vi "LM79 Stabilization.vi"(8 "error in (no error)":errorcluster, 10 "Time Between\nMeasurements (s)":dbl, 11 "Data over time":dbl[](array[numeric])) -> (0 "error out":errorcluster, 1 "Stabilization Data":T1, 2 "Stabilized":bool)   [LabVIEW 2013]
uses:
  MR 16 teardown/MR16TestStandDAQ/Controls/Stabilization.ctl
  <vilib>/Analysis/baseanly.llb/Mean (DBL).vi
  <vilib>/Analysis/NI_AALBase.lvlib
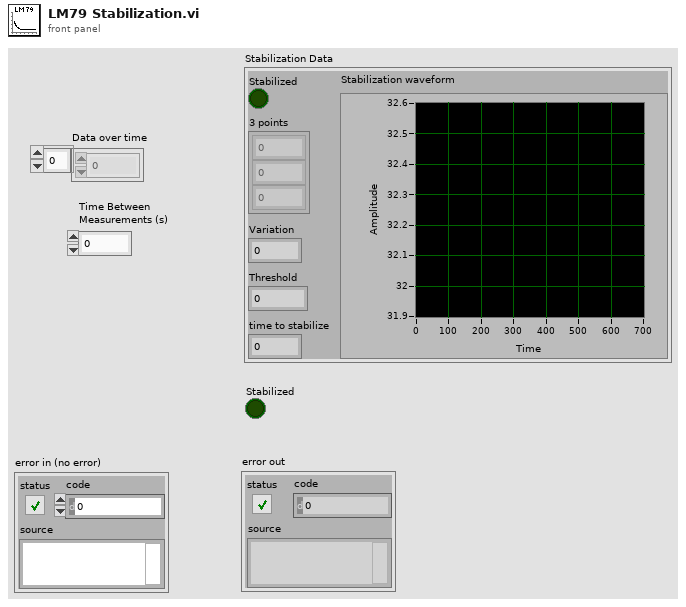
[diagram p1: front panel]
types:
  T1 = typedef "Stabilization.ctl" = cluster{"Stabilization waveform":waveform(dbl), "Variation":dbl, "Stabilized":bool, "Threshold":dbl, "time to stabilize":dbl, "3 points":dbl[]}
  T2 = cluster{waveform(dbl), dbl, bool, dbl, dbl, dbl[]}
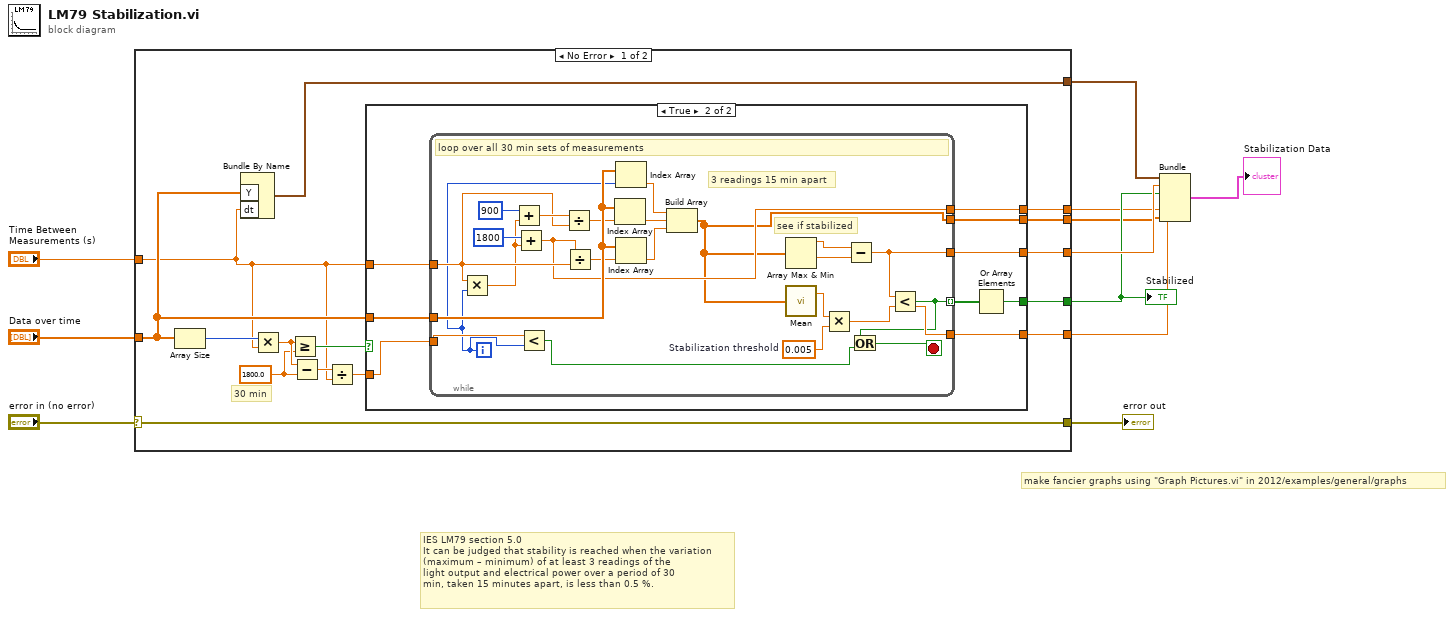
[diagram p0: block diagram]
diagram:
  # "make fancier graphs using \"Graph Pictures.vi\" in 2012/examples/general/graphs"
  # "IES LM79 section 5.0\nIt can be judged that stability is reached when the variation\n(maximum – minimum) of at least 3 readings of the\nlight output and electrical power over a period of 30\nmin, taken 15 minutes apart, is less than 0.5 %."
  n1 = case shown="No Error" "error in (no error)" {
    selector: "error in (no error)" -> [w26 w60]
    tunnel: [w26 w60] -> w10
    tunnel: "Data over time" -> [w21 _]
    tunnel: "Time Between\nMeasurements (s)" -> [w14 _]
    tunnel: [w24 _] -> w7
    tunnel: [w23 _] -> w5
    tunnel: [w16 _] -> w6
    tunnel: [w15 _] -> w4
    tunnel: [w13 _] -> w3
    tunnel: [w12 _] -> w2
    frame No Error {
      w19 = 1800.0 ("y")
      # "30 min"
      n2 = Array Size(array=w21) -> (size(s)=w22:i32)
      n3 = Bundle By Name("Y"=w21, "dt"=w14) -> (w24:waveform(dbl))  [unwired: 1 in]
      n4 = Multiply(x=w22, y=w14) -> (x*y=w20:dbl)
      n5 = Greater Or Equal?(x=w20, y=w19) -> (x >= y?=w25:bool)
      n6 = Subtract(x=w20, y=w19) -> (x-y=w18:dbl)
      n7 = Divide(x=w18, y=w14) -> (x/y=w17:dbl)
      n8 = case shown="True" w25 {
        tunnel: [_ w32] -> w23
        tunnel: w21 -> [_ w35]
        tunnel: w17 -> [_ w29]
        tunnel: w14 -> [_ w34]
        tunnel: [_ w31] -> w16
        tunnel: [_ w30] -> w15
        tunnel: [_ w28] -> w13
        tunnel: [_ w27] -> w12
        frame False {
        }
        frame True {
          n9 = while {
            tunnel: [w39] -> w33 mode=indexing
            tunnel: w35 -> [w55]
            tunnel: w34 -> [w48]
            tunnel: [w45] -> w31
            tunnel: [w44] -> w30
            tunnel: w29 -> [w42]
            tunnel: [w37] -> w28
            tunnel: [w36] -> w27
            i -> [w41]
            stop <- w43 stop-if-true
            w56 = 0.005  # Stabilization threshold
            # "3 readings 15 min apart"
            # "see if stabilized"
            # "loop over all 30 min sets of measurements"
            n10 = Multiply(x=w48, y=w41) -> (x*y=w38:dbl)
            n11 = Add(x=900, y=w38) -> (x+y=w50:dbl)
            n12 = Add(x=1800, y=w38) -> (x+y=w37:dbl)
            n13 = Less?(x=w42, y=w41) -> (x < y?=w40:bool)
            n14 = Divide(x=w50, y=w48) -> (x/y=w46:dbl)
            n15 = Divide(x=w37, y=w48) -> (x/y=w47:dbl)
            n16 = Index Array(array=w55, index=w46) -> (element=w53:dbl)
            n17 = Index Array(array=w55, index=w41) -> (element=w54:dbl)
            n18 = Index Array(array=w55, index=w47) -> (element=w52:dbl)
            n19 = Build Array(w54, w53, w52) -> (w36:dbl[])
            n20 = Array Max & Min(array=w36) -> (max value=w59:dbl, min value=w58:dbl)  [unwired: 2 out]
            n21 = call-poly <vilib>:"Mean.vi"("X"=w36) -> ("mean"=w57:dbl)  [unwired: 1 out]
            n22 = Multiply(x=w57, y=w56) -> (x*y=w44:dbl)
            n23 = Subtract(x=w59, y=w58) -> (x-y=w45:dbl)
            n24 = Less?(x=w45, y=w44) -> (x < y?=w39:bool)
            n25 = Or(x=w39, y=w40) -> (x .or. y?=w43:bool)
          }
          n26 = Or Array Elements(Boolean array=w33) -> (logical OR=w32:bool)
        }
      }
    }
    frame Error {
    }
  }
  "error out" <- w10
  "Stabilized" <- w5
  n27 = Bundle(w7, w6, w5, w4, w3, w2) -> (→"Stabilization Data":T2)  [unwired: 1 in]
